vi "Handle Error.vi"(8 "error in (no error)":errorcluster, 11 "Application in":refnum<class "Application.lvclass">) -> (0 "error out":errorcluster, 3 "Application out":refnum<class "Application.lvclass">)   [LabVIEW 2010, in "Application.lvclass"]
doc: "Handle Error.vi is called after Shutdown.vi. It is called at a point downstream where it can see any error originating in Setup, Execute or Shutdown. It does not see any error that was passed into Run -- in other words, it only sees errors generated by this application. Child classes may override this VI to do error logging, throw error dialogs or other actions appropriate when their application has an unclean exit. Handle Error.vi does not have any way to restart the application. It is for error management only."
uses:
  Application.lvclass
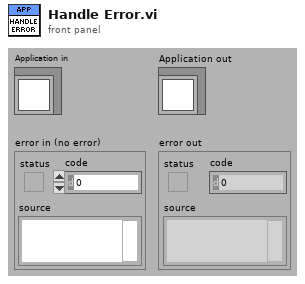
[diagram p1: front panel]
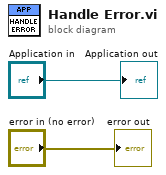
[diagram p0: block diagram]
diagram:
  "error out" <- "error in (no error)"
  "Application out" <- "Application in"
